vi "runHTOutcounterOnly.vi"() -> ()   [LabVIEW 2012]
panel:
  out "appended path":path
  in  "path":path
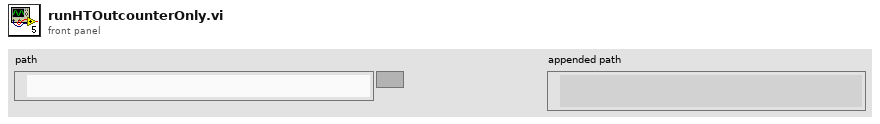
[diagram p1: front panel]
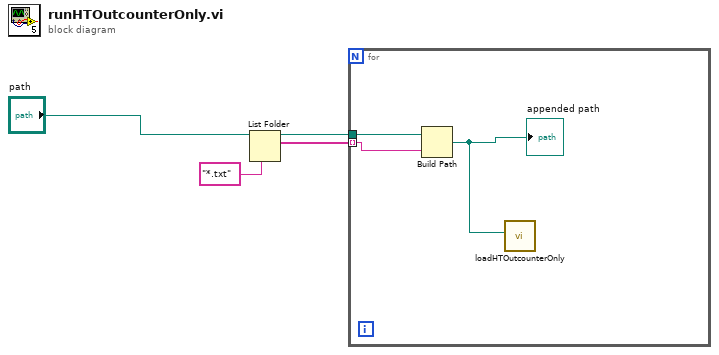
[diagram p0: block diagram]
diagram:
  n1 = List Folder(path="path", pattern="*.txt") -> (path out=w1:path, filenames=w2:string[])  [unwired: 2 in, 2 out]
  n2 = for {
    tunnel: w2 -> [w7] mode=indexing
    tunnel: w1 -> [w6]
    n3 = Build Path(base path=w6, name or relative path=w7) -> (appended path=w5:path)
    "appended path" <- w5
    n4 = call "loadHTOutcounterOnly.vi"("file path (dialog if empty)"=w5) -> ()  [unwired: 11 in]
  }
